vi "To CSV File.vi"(8 "error in (no error)":errorcluster, 9 "Path":path, 10 "engine configuration":refnum<class "engine configuration.lvclass">, 11 "Add Module editor node in":refnum<class "Add Module editor node.lvclass">) -> (0 "error out":errorcluster, 3 "Add Module editor node out":refnum<class "Add Module editor node.lvclass">)   [LabVIEW 2018, in "Add Module editor node.lvclass"]
uses:
  Add Module editor node.lvclass
  <vilib>/NI/Module Execution Interface/Engine Configuration/engine configuration.lvclass
  module/configuration/Add Module configuration.lvclass
  C:/Program Files (x86)/National Instruments/LabVIEW 2018/vi.lib/NI/Configuration Framework/serializable configuration/NISE_CEF_serializable configuration.lvclass
  <vilib>/NI/Configuration Framework/serializable configuration/NISE_CEF_serializable configuration.lvclass/NISE_CEF_serializable configuration.ctl
  module/configuration/Add Module configuration.lvclass/Add Module configuration.ctl
  <vilib>/NI/Tag Bus/tag/tag descriptor.lvclass/tag descriptor.ctl
  <vilib>/Utility/LVClass/Get LV Class Name.vi
  <vilib>/NI/Configuration Framework/error generator/NISE_error generator.vi
  <vilib>/NI/Tag Bus Module Framework/channel/TBM channel.lvclass
  <vilib>/NI/Configuration Framework/serializable configuration/NISE_CEF_serializable configuration.lvclass
  <vilib>/NI/Tag Bus/tag/tag descriptor.lvclass
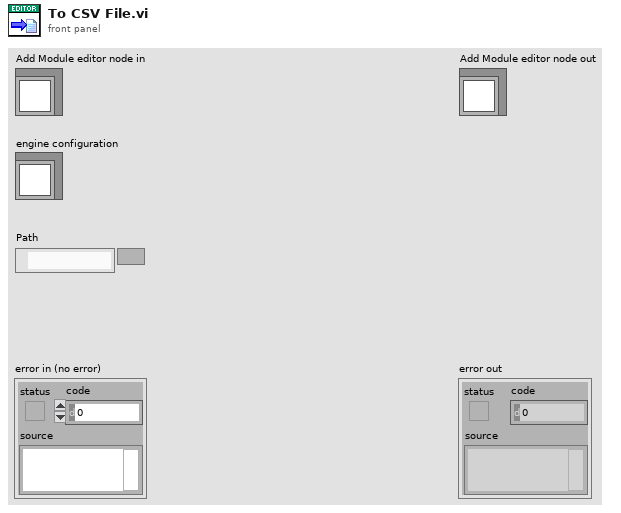
[diagram p1: front panel]
types:
  T1 = typedef "Add Module configuration.lvclass/Line.ctl" = cluster{"channel":refnum<class "TBM channel.lvclass">}
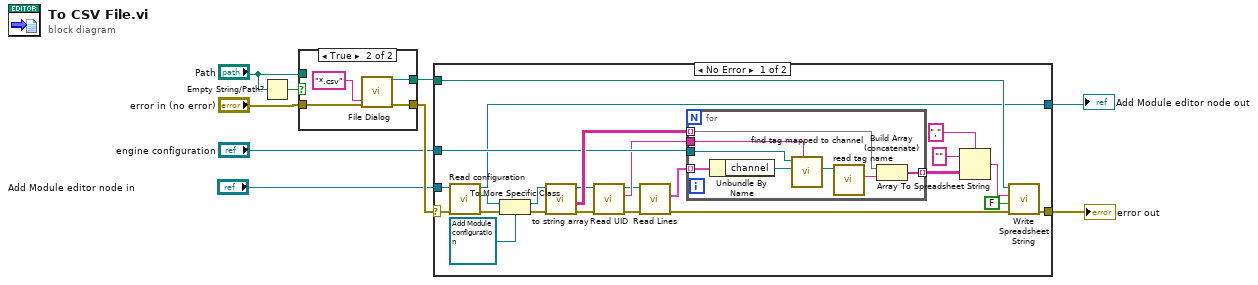
[diagram p0: block diagram]
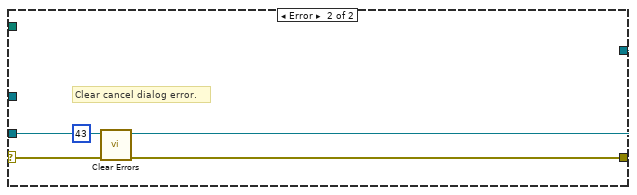
[diagram p3: hidden frame]
diagram:
  n1 = Empty String/Path?(string/path="Path") -> (empty?=w9:bool)
  n2 = case shown="True" w9 {
    tunnel: "error in (no error)" -> [w10 w14]
    tunnel: [w10 w13] -> w7
    tunnel: [w11 w12] -> w8
    tunnel: "Path" -> [w11 _]
    frame False {
    }
    frame True {
      n3 = call "File Dialog"("error in"=w14, "pattern (all files)"="*.csv") -> ("selected path"=w12:path, "error out"=w13:errorcluster)  [unwired: 10 in, 2 out]
    }
  }
  n4 = case shown="No Error" w7 {
    selector: w7 -> [w26 w50]
    tunnel: [w37 w49] -> w2
    tunnel: [w25 w51] -> w1
    tunnel: "Add Module editor node in" -> [w27 w51]
    tunnel: w8 -> [w33 _]
    tunnel: "engine configuration" -> [w30 _]
    frame No Error {
      n5 = call-dynamic "Read configuration.vi"("error in"=w26, "Add Module editor node in"=w27) -> ("error out"=w24:errorcluster, "configuration"=w23:refnum<class "NISE_CEF_serializable configuration.lvclass">, "Add Module editor node out"=w25:refnum<class "Add Module editor node.lvclass">)  [unwired: 7 in]
      n6 = To More Specific Class(target class=refnum<class "Add Module configuration.lvclass"> refnum ("tag bus configurable plugin module configuration"), reference=w23, error in=w24) -> (specific class reference=w39:refnum<class "Add Module configuration.lvclass">, error out=w38:errorcluster)
      n7 = call-dynamic "to string array.vi"("error in (no error)"=w38, "Add Module configuration in"=w39) -> ("error out"=w21:errorcluster, "Array"=w32:string[][], "Add Module configuration out"=w22:refnum<class "Add Module configuration.lvclass">)  [unwired: 6 in, 1 out]
      n8 = call <vilib>:"Read UID.vi"("error in"=w21, "configuration in"=w22) -> ("error out"=w19:errorcluster, "instance id"=w29:string, "configuration out"=w16:refnum<class "Add Module configuration.lvclass">)  [unwired: 7 in]
      n9 = call "Read Lines.vi"("error in (no error)"=w19, "Add Module configuration in"=w16) -> ("error out"=w18:errorcluster, "Lines"=w17:T1[])  [unwired: 7 in, 1 out]
      n10 = for {
        tunnel: w32 -> [w43] mode=indexing
        tunnel: [w41] -> w31 mode=indexing
        tunnel: w17 -> [w47] mode=indexing
        tunnel: w30 -> [w45]
        tunnel: w29 -> [w40]
        n11 = Unbundle By Name(w47) -> ("channel"=w46:refnum<class "TBM channel.lvclass">)
        n12 = call <vilib>:"find tag mapped to channel.vi"("owner"=w40, "channel"=w46, "engine configuration in"=w45) -> ("tag"=w44:refnum<class "tag descriptor.lvclass">)  [unwired: 6 in, 2 out]
        n13 = call <vilib>:"read tag name.vi"("system tag in"=w44) -> ("name"=w42:string)  [unwired: 8 in, 2 out]
        n14 = Build Array (concatenate)(w43, w42) -> (w41:string[])
      }
      n15 = Array To Spreadsheet String(delimiter (Tab)=",", array=w31, 3:"" ("format string")) -> (spreadsheet string=w36:string)
      n16 = call <vilib>:"Write Spreadsheet String.vi"("error in"=w18, "append to file? (new file:F)"=FALSE, "spreadsheet string"=w36, "file path (dialog if empty)"=w33) -> ("error out"=w37:errorcluster)  [unwired: 6 in, 1 out]
    }
    frame Error {
      # "Clear cancel dialog error."
      n17 = call <vilib>:"Clear Errors.vi"("error in (no error)"=w50, "specific error code to clear (0: all)"=43) -> ("error out"=w49:errorcluster)  [unwired: 4 in, 1 out]
    }
  }
  "error out" <- w2
  "Add Module editor node out" <- w1
